vi "Stepper PWM.vi"(0 "Drive Pin 2":refnum<k21>, 1 "Drive Pin 1":refnum<k21>, 2 "Duty Cycle (0-1999)":u16) -> ()   [LabVIEW 2019]
uses:
  <vilib>/rvi/eio/common/nirviEmuTemplateMethod_errors.vi
  <vilib>/eio/EIONode/EIONode.xnode
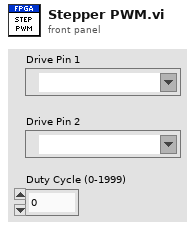
[diagram p1: front panel]
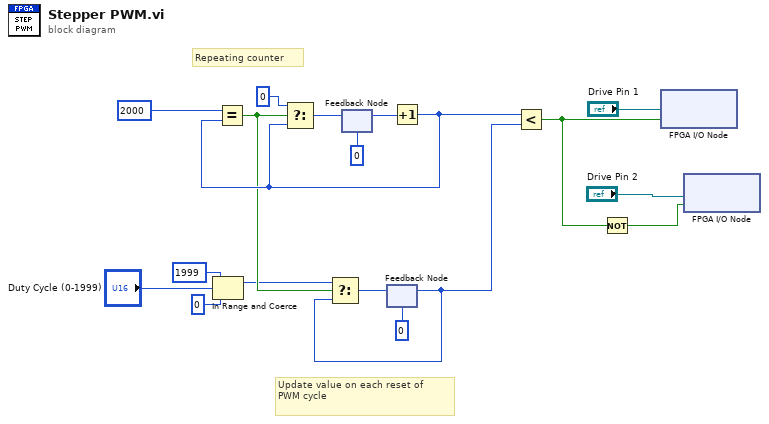
[diagram p0: block diagram]
diagram:
  # "Repeating counter"
  # "Update value on each reset of \nPWM cycle"
  n1 = In Range and Coerce(upper limit=u16 1999, x="Duty Cycle (0-1999)", lower limit=u16 0) -> (coerced(x)=w5:u16)  [unwired: 1 out]
  n2 = feedback #1(u16 0 ("Compare Value")) -> (w13:u16)
  n3 = feedback #2(u16 0 ("Compare Value")) -> (w9:u16)
  n4 = Increment(x=w13) -> (x+1=w10:u16)
  n5 = Equal?(x=u16 2000 ("Period"), y=w10) -> (x = y?=w8:bool)
  n6 = Select(t=u16 0, s=w8, f=w10) -> (s? t:f=w15:u16)
  n7 = Select(t=w5, s=w8, f=w9) -> (s? t:f=w16:u16)
  n8 = feedback-in #1(w15) -> ()
  n9 = feedback-in #2(w16) -> ()
  n10 = Less?(x=w10, y=w9) -> (x < y?=w1:bool)
  n11 = Not(x=w1) -> (.not. x?=w2:bool)
  n12 = xnode "FPGA I/O Node"("I/O项"=w1, "FPGA I/O输入"="Drive Pin 1") -> ()  [unwired: 1 out]
  n13 = xnode "FPGA I/O Node"("I/O项"=w2, "FPGA I/O输入"="Drive Pin 2") -> ()  [unwired: 1 out]
